vi "Get XY.vi"(8 "error in":errorcluster, 10 "device name":tag) -> (0 "error out":errorcluster, 2 "Y":dbl, 3 "X":dbl)   [LabVIEW 2015]
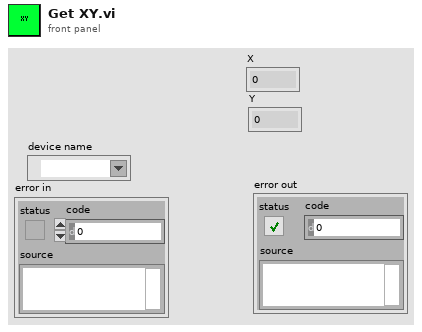
[diagram p1: front panel]
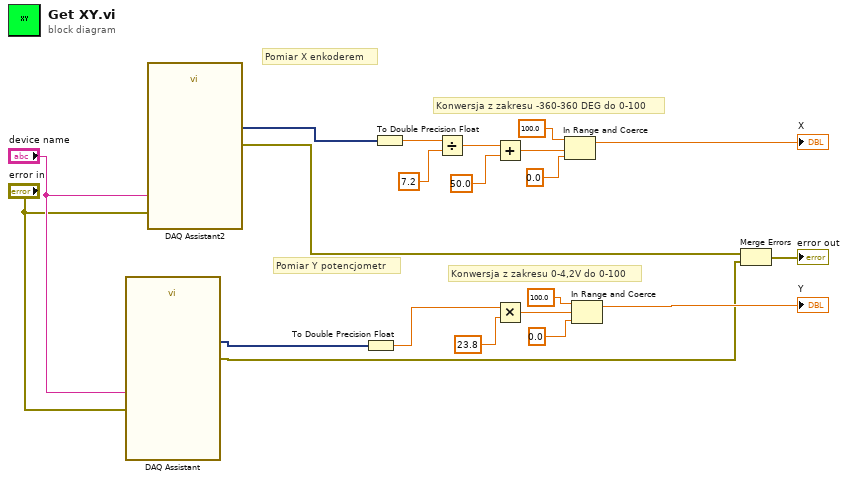
[diagram p0: block diagram]
diagram:
  # "Konwersja z zakresu 0-4,2V do 0-100"
  # "Konwersja z zakresu -360-360 DEG do 0-100"
  # "Pomiar Y potencjometr"
  # "Pomiar X enkoderem"
  n1 = call "DAQ Assistant"("error in"="error in", "device name"="device name") -> ("data"=w6:dynamicdata, "error out"=w5:errorcluster)  [unwired: 15 in, 1 out]
  n2 = call "DAQ Assistant2"("error in"="error in", "device name"="device name") -> ("data"=w1:dynamicdata, "error out"=w2:errorcluster)  [unwired: 14 in, 2 out]
  n3 = To Double Precision Float(number=w6) -> (double precision float=w17:dbl)
  n4 = To Double Precision Float(number=w1) -> (double precision float=w21:dbl)
  n5 = Divide(x=w21, y=7.2) -> (x/y=w19:dbl)
  n6 = Add(x=w19, y=50.0) -> (x+y=w14:dbl)
  n7 = Multiply(x=w17, y=23.8) -> (x*y=w11:dbl)
  n8 = In Range and Coerce(upper limit=100.0, x=w14, lower limit=0.0) -> (coerced(x)=→"X":dbl)  [unwired: 1 out]
  n9 = In Range and Coerce(upper limit=100.0, x=w11, lower limit=0.0) -> (coerced(x)=→"Y":dbl)  [unwired: 1 out]
  n10 = Merge Errors(w2, w5) -> (→"error out":errorcluster)
